vi "Unsubscribe (SingleTopic).vi"(6 "timeout (100ms)":i32=100, 8 "error in (no error)":errorcluster, 10 "Topic Filter":string, 11 "MQTT_Base in":refnum<class "MQTT_Base.lvclass">) -> (0 "error out":errorcluster, 3 "MQTT_Base out":refnum<class "MQTT_Base.lvclass">)   [LabVIEW 2013, in "MQTT Base.lvlib" / "MQTT_Base.lvclass"]
uses:
  MQTT_Base.lvclass
  <vilib>/LabVIEW Open Source Project/MQTT Control Packets/Control Packets/UNSUBSCRIBE/UNSUBSCRIBE.lvclass
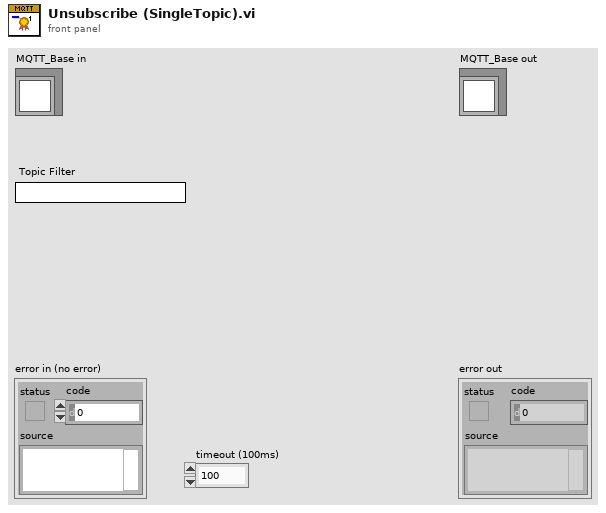
[diagram p1: front panel]
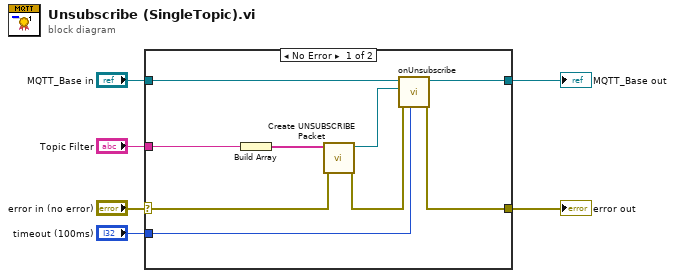
[diagram p0: block diagram]
diagram:
  n1 = case shown="No Error" "error in (no error)" {
    selector: "error in (no error)" -> [w14 w17]
    tunnel: [w9 w17] -> w5
    tunnel: [w8 w16] -> w3
    tunnel: "MQTT_Base in" -> [w12 w16]
    tunnel: "Topic Filter" -> [w13 _]
    tunnel: "timeout (100ms)" -> [w7 _]
    frame No Error {
      n2 = Build Array(w13) -> (w15:string[])
      n3 = call <vilib>:"Create UNSUBSCRIBE Packet.vi"("error in (no error)"=w14, "Topic Subscriptions"=w15) -> ("error out"=w10:errorcluster, "UNSUBSCRIBE out"=w11:refnum<class "UNSUBSCRIBE.lvclass">)  [unwired: 7 in, 1 out]
      n4 = call-dynamic "onUnsubscribe.vi"("timeout (100ms)"=w7, "error in (no error)"=w10, "UNSUBSCRIBE"=w11, "MQTT_Base in"=w12) -> ("error out"=w9:errorcluster, "MQTT_Base out"=w8:refnum<class "MQTT_Base.lvclass">)  [unwired: 5 in, 1 out]
    }
    frame Error {
    }
  }
  "error out" <- w5
  "MQTT_Base out" <- w3
